vi "718_DC Motor_PID_test_3.vi"() -> ()   [LabVIEW 2018]
uses:
  <userlib>/KNR OS 4.0 LabVIEW Toolkit/Type Definition/DC Motor Port.ctl
  <userlib>/KNR OS 4.0 LabVIEW Toolkit/Type Definition/Resource.ctl
panel:
  in  "M2 Reverse":bool
  out "Speed (+-100%)11":dbl
  out "Speed (+-100%) 21":dbl
  in  "Enable Motor 2":bool
  in  "Enable sync":bool=TRUE
  in  "Kp 3":dbl(slide)=0.2 scale=0.0..0.8
  in  "Ki 3":dbl(slide)=0.05 scale=0.0..0.02
  in  "Kd 3":dbl(slide)=0.1 scale=0.0..0.2
  in  "PID sync":bool=TRUE
  out "Speed (+-100%) 22":dbl
  out "Velocity (cm/sec) 2":dbl
  in  "Port 2":T1=5 items=["DS1"=4, "DS2"=5, "DS3"=6, "DS4"=7]
  out "Velocity (cm/sec) Chart 2":dbl(graph)
  out "Desire Velosity (cm/sec) 2":dbl
  in  "Desire Velosity (cm/sec)":dbl=15.0 format="%#_13g"
  in  "F/B switch":bool=TRUE
  in  "Port":T1=4 items=["DS1"=4, "DS2"=5, "DS3"=6, "DS4"=7]
  out "Velocity (cm/sec) Chart":dbl(graph)
  out "Speed (+-100%)12":dbl
  in  "Kd":dbl(slide)=0.1 scale=0.0..0.2
  in  "Ki":dbl(slide)=0.05 scale=0.0..0.05
  in  "Kp":dbl(slide)=0.2 scale=0.0..0.8
  in  "stop":bool
  in  "Enable Motor 1":bool
  out "Velocity (cm/sec)":dbl
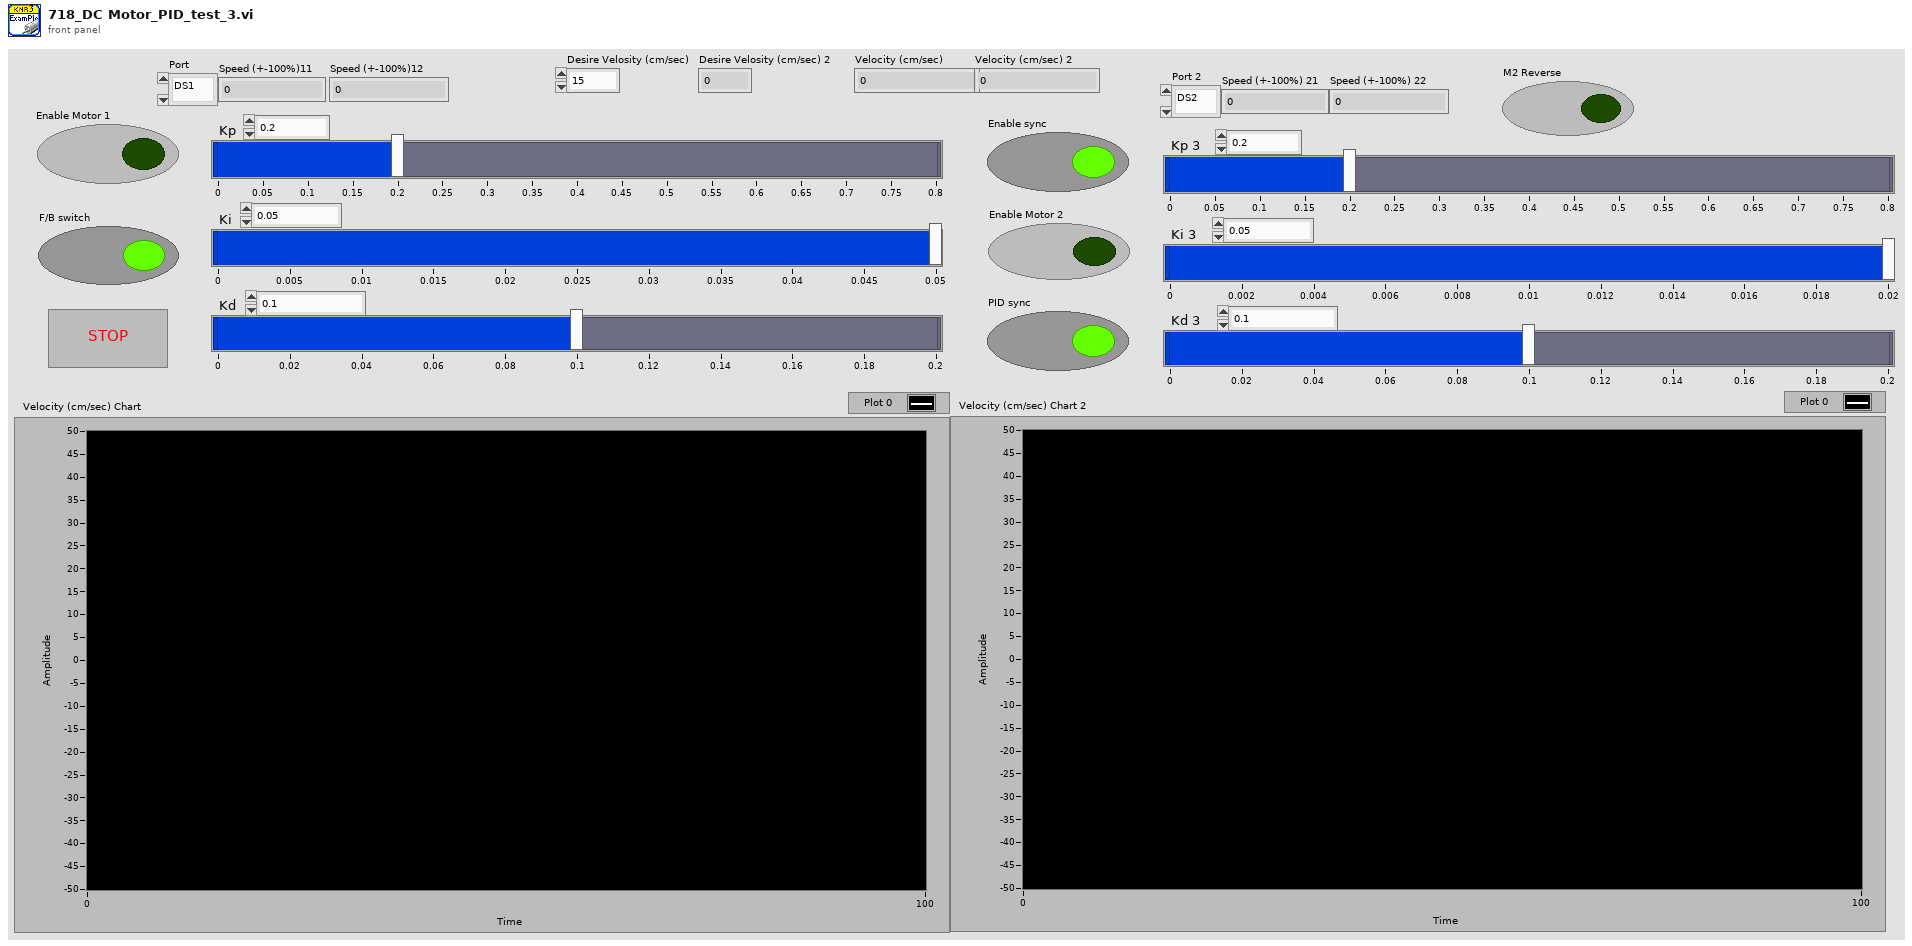
[diagram p1: front panel]
types:
  T1 = typedef "DC Motor Port.ctl" = u16
  T2 = typedef "Resource.ctl" = enum16{"KNRm_DDRC", "KNRm_DDDD", "KNRm_DDDR", "KNRm_DDDC", "KNR", "KNRm_neww"}
  T3 = typedef "KNR3 Reference.ctl" = cluster{"FPGA Session":refnum<class "FPGA Interface Base.lvclass">, "Resource":T2}
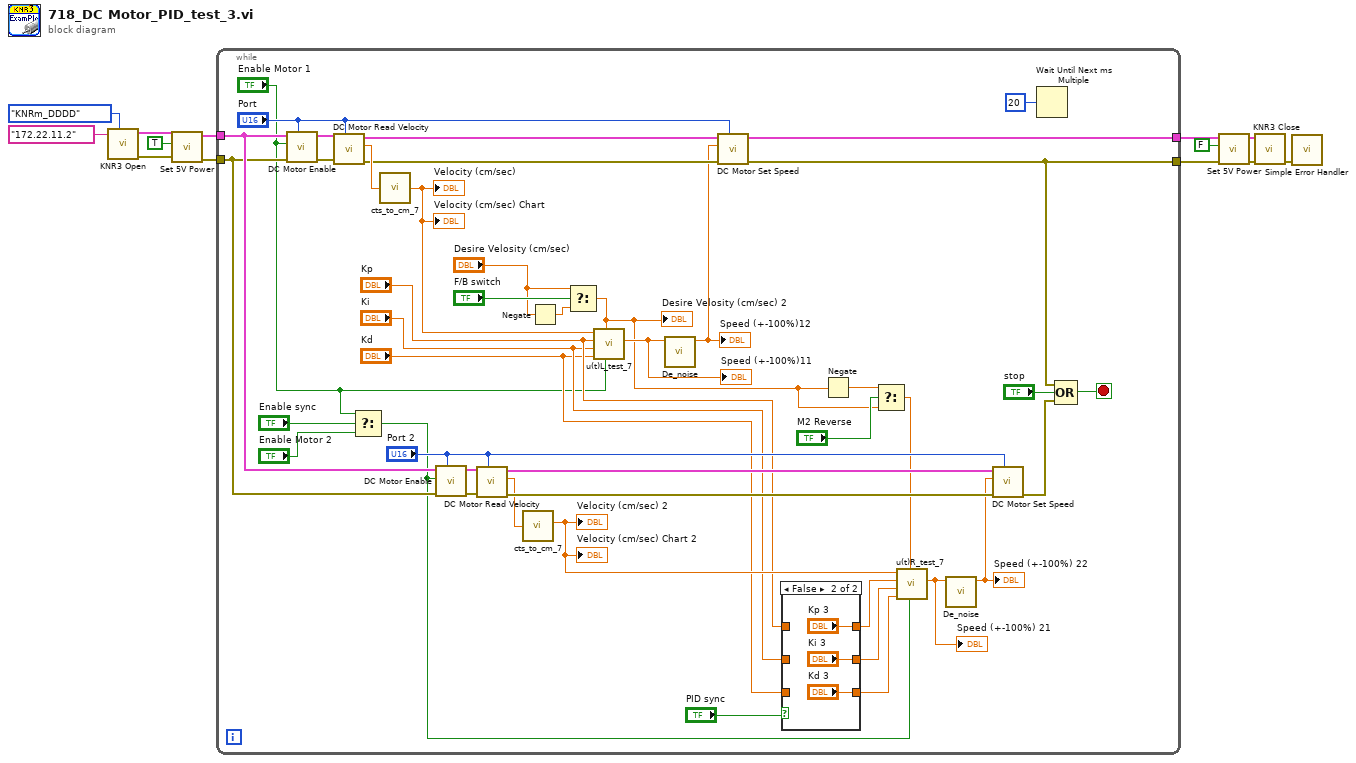
[diagram p0: block diagram]
diagram:
  n1 = call <userlib>:"KNR3 Open.vi"("Resource"=Resource."KNRm_DDDD", "IP"="172.22.11.2") -> ("error out"=w6:errorcluster, "KNR out"=w8:T3)  [unwired: 8 in]
  n2 = call <userlib>:"Set 5V Power.vi"("error in (no error)"=w6, "5V Power(T)"=TRUE ("5V Power"), "KNR in"=w8) -> ("error out"=w10:errorcluster, "KNR out"=w11:T3)  [unwired: 7 in]
  n3 = while {
    tunnel: w11 -> [w38]
    tunnel: w10 -> [w37]
    tunnel: [w49] -> w4
    tunnel: [w48] -> w3
    stop <- w55 stop-if-true
    n4 = call <userlib>:"DC Motor Enable.vi"("Port (DS1)"="Port", "error in (no error)"=w37, "Enable Motor(F)"="Enable Motor 1", "KNR in"=w38) -> ("error out"=w52:errorcluster, "KNR out"=w53:T3)  [unwired: 6 in]
    n5 = call <userlib>:"DC Motor Read Velocity.vi"("Port (DS1)"="Port", "error in (no error)"=w52, "KNR in"=w53) -> ("error out"=w45:errorcluster, "Velocity (cts/sec)"=w51:dbl, "KNR out"=w46:T3)  [unwired: 6 in]
    n6 = Select(t="Enable Motor 1", s="Enable sync", f="Enable Motor 2") -> (s? t:f=w24:bool)
    n7 = call "cts_to_cm_7.vi"("cts"=w51) -> ("cm"=w31:dbl)
    "Velocity (cm/sec)" <- w31
    "Velocity (cm/sec) Chart" <- w31
    n8 = call <userlib>:"DC Motor Enable.vi"("Port (DS1)"="Port 2", "error in (no error)"=w37, "Enable Motor(F)"=w24, "KNR in"=w38) -> ("error out"=w40:errorcluster, "KNR out"=w39:T3)  [unwired: 6 in]
    n9 = call <userlib>:"DC Motor Read Velocity.vi"("Port (DS1)"="Port 2", "error in (no error)"=w40, "KNR in"=w39) -> ("error out"=w44:errorcluster, "Velocity (cts/sec)"=w41:dbl, "KNR out"=w43:T3)  [unwired: 6 in]
    n10 = call "cts_to_cm_7.vi"("cts"=w41) -> ("cm"=w33:dbl)
    "Velocity (cm/sec) 2" <- w33
    "Velocity (cm/sec) Chart 2" <- w33
    n11 = Negate(x="Desire Velosity (cm/sec)") -> (-x=w21:dbl)
    n12 = Select(t="Desire Velosity (cm/sec)", s="F/B switch", f=w21) -> (s? t:f=w14:dbl)
    "Desire Velosity (cm/sec) 2" <- w14
    n13 = call "u(t)L_test_7.vi"("enable"="Enable Motor 1", "Desire Velosity"=w14, "Kd"="Kd", "Ki"="Ki", "Kp"="Kp", "Velocity"=w31) -> ("u(t)"=w47:dbl)  [unwired: 5 in]
    "Speed (+-100%)11" <- w47
    n14 = call "De_noise.vi"("u(t)"=w47) -> ("u(t)2"=w19:dbl)  [unwired: 10 in]
    "Speed (+-100%)12" <- w19
    n15 = call <userlib>:"DC Motor Set Speed.vi"("Port (DS1)"="Port", "error in (no error)"=w45, "Speed (+-100%)"=w19, "KNR in"=w46) -> ("error out"=w48:errorcluster, "KNR out"=w49:T3)  [unwired: 6 in]
    n16 = case shown="False" "PID sync" {
      tunnel: [w59 "Kp 3"] -> w36
      tunnel: [w57 "Kd 3"] -> w35
      tunnel: [w58 "Ki 3"] -> w34
      tunnel: "Kp" -> [w59 _]
      tunnel: "Ki" -> [w58 _]
      tunnel: "Kd" -> [w57 _]
      frame True {
      }
      frame False {
      }
    }
    n17 = Negate(x=w14) -> (-x=w13:dbl)
    n18 = Select(t=w13, s="M2 Reverse", f=w14) -> (s? t:f=w16:dbl)
    n19 = call "u(t)R_test_7.vi"("enable"=w24, "Desire Velosity"=w16, "Kd"=w35, "Ki"=w34, "Kp"=w36, "Velocity"=w33) -> ("u(t)"=w17:dbl)  [unwired: 5 in]
    "Speed (+-100%) 21" <- w17
    n20 = call "De_noise.vi"("u(t)"=w17) -> ("u(t)2"=w18:dbl)  [unwired: 10 in]
    "Speed (+-100%) 22" <- w18
    n21 = call <userlib>:"DC Motor Set Speed.vi"("Port (DS1)"="Port 2", "error in (no error)"=w44, "Speed (+-100%)"=w18, "KNR in"=w43) -> ("error out"=w20:errorcluster)  [unwired: 6 in, 1 out]
    n22 = Wait Until Next ms Multiple(millisecond multiple=u32 20) -> ()  [unwired: 1 out]
    n23 = Compound Arithmetic op=OR(w48, "stop", w20) -> (w55:bool)
  }
  n24 = call <userlib>:"Set 5V Power.vi"("5V Power(T)"=FALSE, "KNR in"=w4) -> ("KNR out"=w2:T3)  [unwired: 8 in, 1 out]
  n25 = call <userlib>:"KNR3 Close.vi"("error in (no error)"=w3, "KNR in"=w2) -> ("error out"=w9:errorcluster)  [unwired: 9 in]
  n26 = call <vilib>:"Simple Error Handler.vi"("error in (no error)"=w9) -> ()  [unwired: 4 in, 5 out]
